vi "Write Auto update indicator.vi"(8 "error in (no error)":errorcluster, 10 "Auto update indicator":bool, 11 "D_Datagrid in":refnum<class "D_Datagrid.lvclass">) -> (0 "error out":errorcluster, 3 "D_Datagrid out":refnum<class "D_Datagrid.lvclass">)   [LabVIEW 2018, in "D Datagrid Library.lvlib" / "D_Datagrid.lvclass"]
uses:
  D_Datagrid.lvclass
  D_Datagrid.lvclass/D_Datagrid.ctl
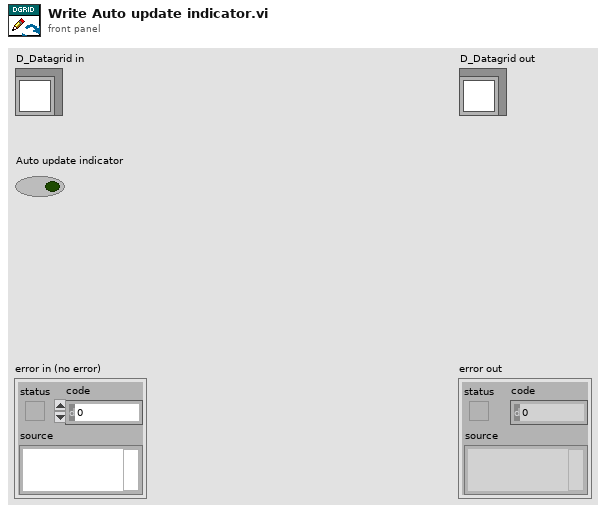
[diagram p1: front panel]
types:
  T1 = typedef "D Datagrid Library.lvlib/D_Datagrid.lvclass/State Data.ctl" = cluster{"Data elements":refnum<class "DatagridElement.lvclass">[][], "Auto-update indicator":bool}
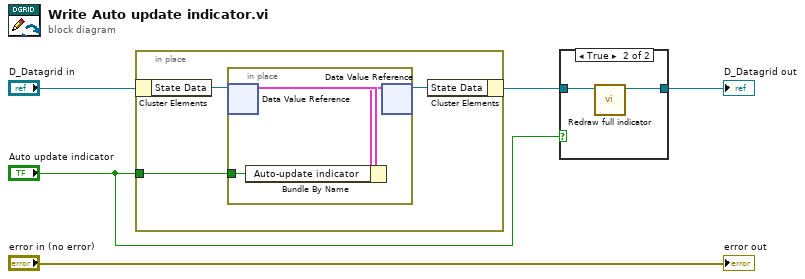
[diagram p0: block diagram]
diagram:
  n1 = in-place {
    in-place-border: "Auto update indicator" -> [w7]
    n2 = in-place-cluster #1("D_Datagrid in") -> ("State Data"=w8:refnum<data-value>)
    n3 = in-place {
      in-place-border: w7 -> [w11]
      n4 = in-place-dvr #2(w8) -> (w10:T1)  [unwired: 1 out]
      n5 = Bundle By Name(cluster=w10, "Auto-update indicator"=w11) -> (w9:T1)
      n6 = in-place-dvr #2(w9) -> (w6:refnum<data-value>)  [unwired: 1 out]
    }
    n7 = in-place-cluster #1("State Data"=w6) -> (w4:refnum<class "D_Datagrid.lvclass">)
  }
  n8 = case shown="True" "Auto update indicator" {
    tunnel: w4 -> [w12 w14]
    tunnel: [w12 w13] -> w3
    frame False {
    }
    frame True {
      n9 = call "Redraw full indicator.vi"("D_Datagrid in"=w14) -> ("D_Datagrid out"=w13:refnum<class "D_Datagrid.lvclass">)  [unwired: 9 in, 1 out]
    }
  }
  "D_Datagrid out" <- w3
  "error out" <- "error in (no error)"
